vi "7Segment.vi"() -> ()   [LabVIEW 2020]
panel:
  in  "Slide":dbl(slide) scale=0.0..70.0
  out "?":bool
  out "?":bool
  out "?":bool
  out "B":bool
  out "?":bool
  out "?":bool
  out "A":bool
  in  "stop":bool
  out "?":bool
  out "?":bool
  out "?":bool
  out "B":bool
  out "?":bool
  out "?":bool
  out "A":bool
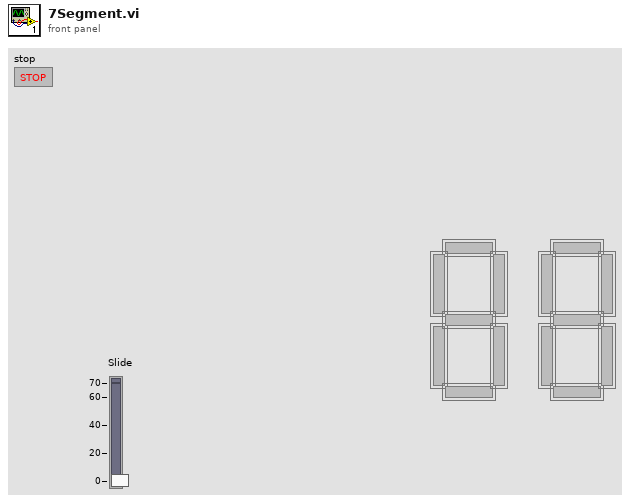
[diagram p1: front panel]
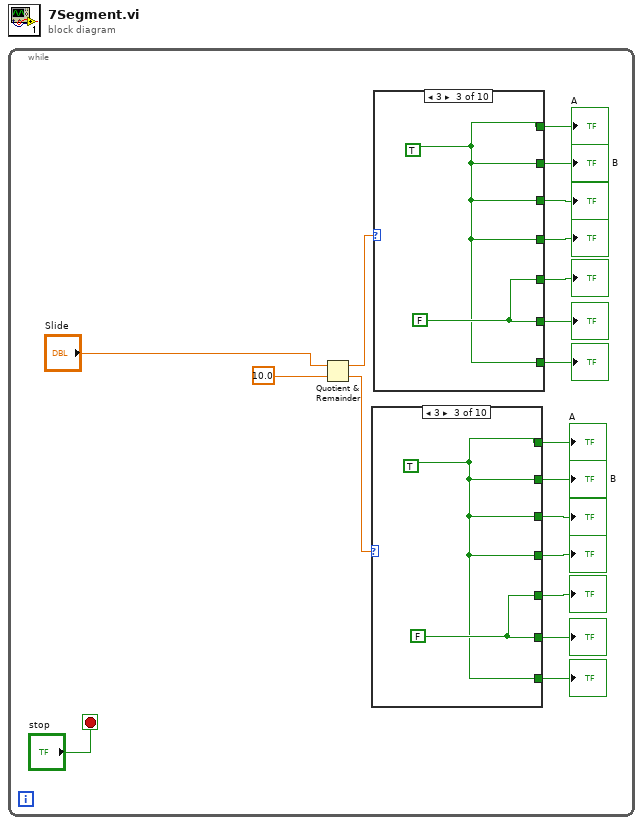
[diagram p0: block diagram]
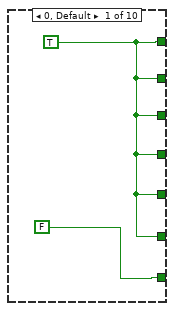
[diagram p2: hidden frame]
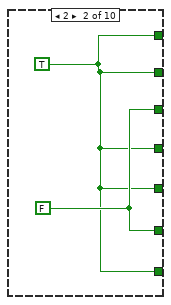
[diagram p3: hidden frame]
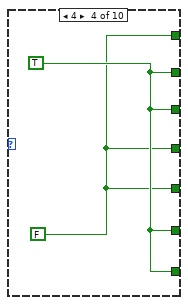
[diagram p4: hidden frame]
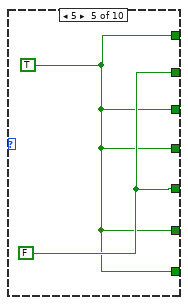
[diagram p5: hidden frame]
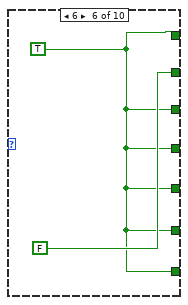
[diagram p6: hidden frame]
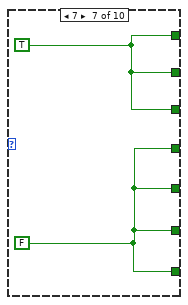
[diagram p7: hidden frame]
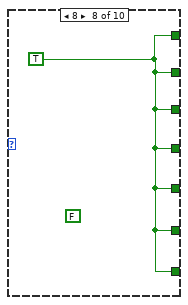
[diagram p8: hidden frame]
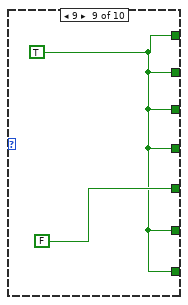
[diagram p9: hidden frame]
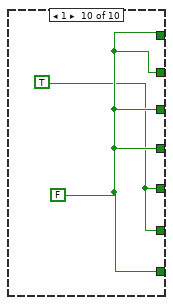
[diagram p10: hidden frame]
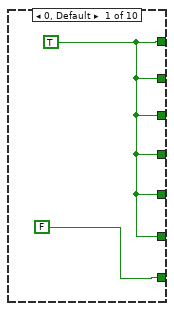
[diagram p11: hidden frame]
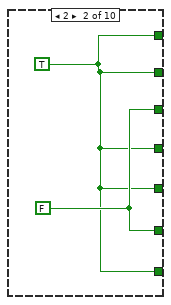
[diagram p12: hidden frame]
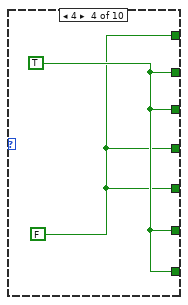
[diagram p13: hidden frame]
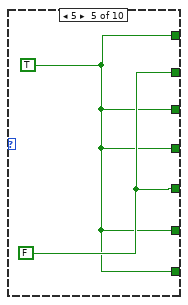
[diagram p14: hidden frame]
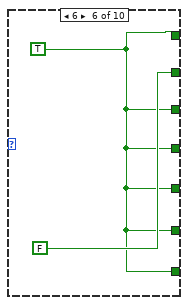
[diagram p15: hidden frame]
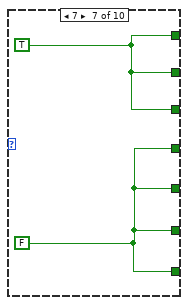
[diagram p16: hidden frame]
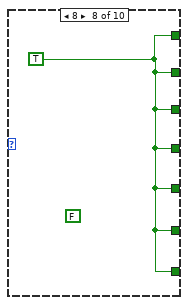
[diagram p17: hidden frame]
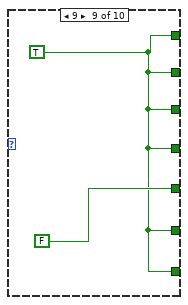
[diagram p18: hidden frame]
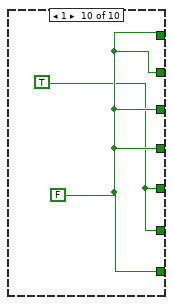
[diagram p19: hidden frame]
diagram:
  n1 = while {
    stop <- "stop" stop-if-true
    n2 = Quotient & Remainder(x="Slide", y=10.0) -> (x-y*floor(x/y)=w3:dbl, floor(x/y)=w2:dbl)
    n3 = case shown="3" w2 {
      tunnel: [w21 w22 w24 w26 w28 w30 w33 w34 w35 w38] -> w11
      tunnel: [w21 w22 w24 w27 w29 FALSE w33 w34 w35 w38] -> w10
      tunnel: [w21 w23 w24 w27 w28 w30 w33 w34 w35 w38] -> w9
      tunnel: [w21 w22 w24 w26 w28 w30 w32 w34 w35 w38] -> w8
      tunnel: [w21 w22 w25 w26 w29 w30 w32 w34 FALSE w37] -> w7
      tunnel: [w21 w23 w25 w27 w28 w30 w32 w34 w35 w37] -> w6
      tunnel: [FALSE w22 w24 w27 w28 w30 w32 w34 w35 w38] -> w5
      frame 0, Default {
        w21 = TRUE
      }
      frame 2 {
        w23 = FALSE
        w22 = TRUE
      }
      frame 3 {
        w25 = FALSE
        w24 = TRUE
      }
      frame 4 {
        w26 = FALSE
        w27 = TRUE
      }
      frame 5 {
        w29 = FALSE
        w28 = TRUE
      }
      frame 6 {
        w30 = TRUE
      }
      frame 7 {
        w32 = FALSE
        w33 = TRUE
      }
      frame 8 {
        (unwired) FALSE
        w34 = TRUE
      }
      frame 9 {
        w35 = TRUE
      }
      frame 1 {
        w38 = FALSE
        w37 = TRUE
      }
    }
    "A" <- w11
    "?" <- w6
    "?" <- w7
    "B" <- w10
    "?" <- w5
    "?" <- w8
    "?" <- w9
    n4 = case shown="3" w3 {
      tunnel: [w40 w41 w43 w45 w47 w49 w52 w53 w54 w57] -> w18
      tunnel: [w40 w41 w43 w46 w48 FALSE w52 w53 w54 w57] -> w17
      tunnel: [w40 w42 w43 w46 w47 w49 w52 w53 w54 w57] -> w16
      tunnel: [w40 w41 w43 w45 w47 w49 w51 w53 w54 w57] -> w15
      tunnel: [w40 w41 w44 w45 w48 w49 w51 w53 FALSE w56] -> w14
      tunnel: [w40 w42 w44 w46 w47 w49 w51 w53 w54 w56] -> w13
      tunnel: [FALSE w41 w43 w46 w47 w49 w51 w53 w54 w57] -> w12
      frame 0, Default {
        w40 = TRUE
      }
      frame 2 {
        w42 = FALSE
        w41 = TRUE
      }
      frame 3 {
        w44 = FALSE
        w43 = TRUE
      }
      frame 4 {
        w45 = FALSE
        w46 = TRUE
      }
      frame 5 {
        w48 = FALSE
        w47 = TRUE
      }
      frame 6 {
        w49 = TRUE
      }
      frame 7 {
        w51 = FALSE
        w52 = TRUE
      }
      frame 8 {
        (unwired) FALSE
        w53 = TRUE
      }
      frame 9 {
        w54 = TRUE
      }
      frame 1 {
        w57 = FALSE
        w56 = TRUE
      }
    }
    "A" <- w18
    "?" <- w13
    "?" <- w14
    "B" <- w17
    "?" <- w12
    "?" <- w15
    "?" <- w16
  }
